vi "Vector A to B.vi"(1 "destination":cluster{"x":dbl, "y 2":dbl}, 2 "Current":T1) -> (0 "vector":cluster{dbl, "Bearing":dbl})   [LabVIEW 2017]
uses:
  040-typeDefs/Position.ctl
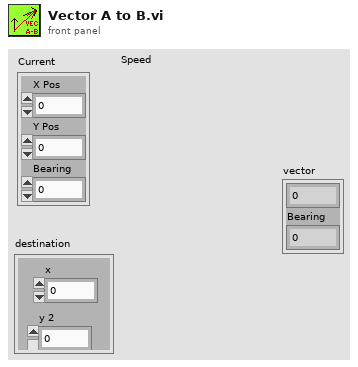
[diagram p1: front panel]
types:
  T1 = typedef "Position.ctl" = cluster{"X Pos":dbl, "Y Pos":dbl, "Bearing":dbl}
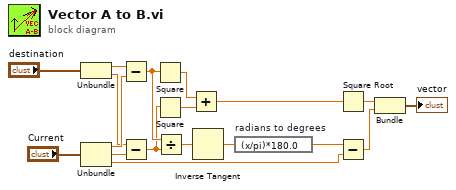
[diagram p0: block diagram]
diagram:
  n1 = Unbundle("destination") -> ("x"=w17:dbl, "y 2"=w15:dbl)
  n2 = Unbundle("Current") -> ("X Pos"=w16:dbl, "Y Pos"=w14:dbl, "Bearing"=w2:dbl)
  n3 = Subtract(x=w17, y=w16) -> (x-y=w10:dbl)
  n4 = Subtract(x=w15, y=w14) -> (x-y=w9:dbl)
  n5 = Square(x=w10) -> (x^2=w11:dbl)
  n6 = Square(x=w9) -> (x^2=w8:dbl)
  n7 = Divide(x=w10, y=w9) -> (x/y=w13:dbl)
  n8 = Add(x=w11, y=w8) -> (x+y=w7:dbl)
  n9 = Inverse Tangent(1:w13) -> (0:w12:dbl)
  n10 = expression code="(x/pi)*180.0" "radians to degrees"(w12) -> (w3:dbl)
  n11 = Square Root(x=w7) -> (sqrt(x)=w6:dbl)
  n12 = Subtract(x=w3, y=w2) -> (x-y=w1:dbl)
  n13 = Bundle(w6, w1) -> (→"vector":cluster{dbl, dbl})  [unwired: 1 in]
